vi "GetGObjectDetails.vi"(8 "error in (no error)":errorcluster, 11 "GObject":refnum<vi>) -> (0 "error out":errorcluster, 3 "output cluster":T1)   [LabVIEW 2014, in "SmartPalette.lvlib"]
uses:
  SmartPalette.lvlib
  Controls/GObjectDetail.ctl
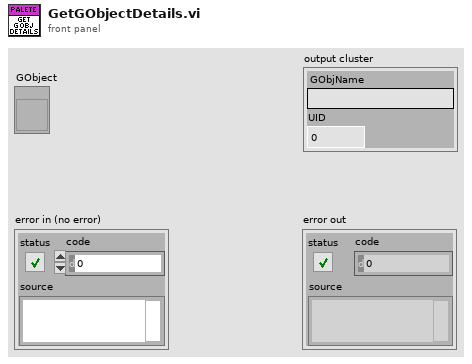
[diagram p1: front panel]
types:
  T1 = typedef "SmartPalette.lvlib/GObjectDetail.ctl" = cluster{"GObjName":string, "UID":i32}
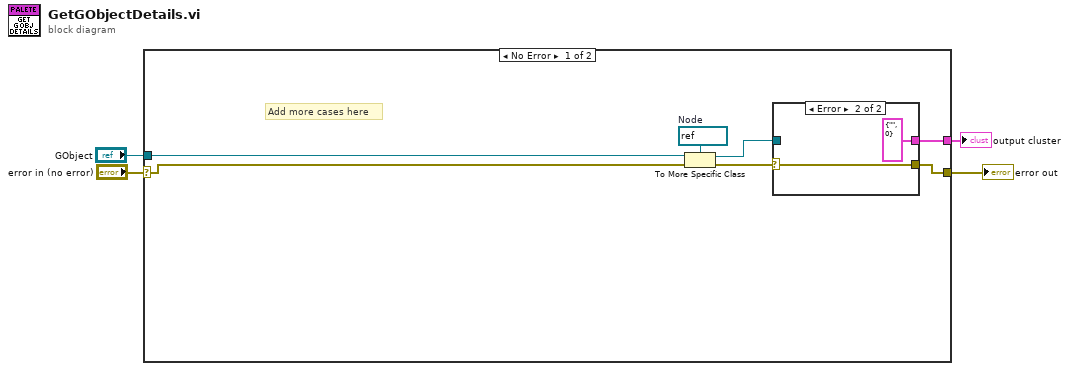
[diagram p0: block diagram]
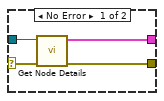
[diagram p2: hidden frame]
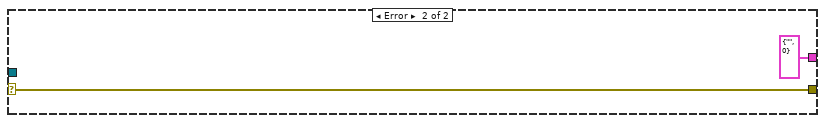
[diagram p3: hidden frame]
diagram:
  n1 = case shown="No Error" "error in (no error)" {
    selector: "error in (no error)" -> [w11 w18]
    tunnel: "GObject" -> [w10 _]
    tunnel: [w7 w18] -> w2
    tunnel: [w5 T1 {"GObjName"="", "UID"=0} ("output cluster")] -> w1
    frame No Error {
      w9 = refnum<vi> refnum  # Node
      # "Add more cases here"
      n2 = To More Specific Class(target class=w9, reference=w10, error in=w11) -> (specific class reference=w6:refnum<vi>, error out=w8:errorcluster)
      n3 = case shown="Error" w8 {
        selector: w8 -> [w15 w17]
        tunnel: [w14 w17] -> w7
        tunnel: w6 -> [w13 _]
        tunnel: [w12 T1 {"GObjName"="", "UID"=0} ("output cluster")] -> w5
        frame No Error {
          n4 = call "Get Node Details.vi"("error in (no error)"=w15, "Node Refnum"=w13) -> ("error out"=w14:errorcluster, "output cluster"=w12:T1)  [unwired: 8 in]
        }
        frame Error {
        }
      }
    }
    frame Error {
    }
  }
  "error out" <- w2
  "output cluster" <- w1
